vi "Main.vi"() -> ()   [LabVIEW 2017]
doc: "The myRIO Project template acquires acceleration data from the onboard accelerometer and displays the changes of acceleration values in a waveform chart."
uses:
  <vilib>/myRIO/Common/Instrument Driver Framework/myRIO v1.0/IRQ/typedefs/DI IRQ Type.ctl
  <vilib>/userdefined/High Color/nirio_resource_hc.ctl
  <vilib>/myRIO/Instrument Drivers/Onboard IO/DIO/typedefs/DIO Reference.ctl
  <vilib>/myRIO/Common/Instrument Driver Framework/Utilities/typedefs/myRIO Generic Hardware Reference.ctl
  <vilib>/myRIO/Common/Instrument Driver Framework/Utilities/typedefs/Hardware Version Enum.ctl
  <vilib>/myRIO/Common/Instrument Driver Framework/Utilities/typedefs/myRIO v1.0 Reference.ctl
  <vilib>/myRIO/Common/Instrument Driver Framework/Utilities/typedefs/Generic FPGA Reference.ctl
  <vilib>/myRIO/Common/Instrument Driver Framework/myRIO v1.0/DIO/typedefs/DIO Channels List.ctl
  <vilib>/myRIO/Common/Instrument Driver Framework/myRIO v1.0/DIO/typedefs/DIO Channels Enum.ctl
  <vilib>/myRIO/Common/Instrument Driver Framework/Utilities/vis/Is FPGA Ref Available.vi
  <vilib>/myRIO/Common/Instrument Driver Framework/myRIO v1.0/DIO/vis/myRIO v1.1 Open DIO.vi
  <vilib>/myRIO/Instrument Drivers/Onboard IO/DIO/vis/Write.vi
  <vilib>/myRIO/Common/Instrument Driver Framework/Utilities/vis/Validate Channels.vi
  <vilib>/myRIO/Common/Instrument Driver Framework/myRIO v1.0/DIO/vis/myRIO v1.0 Reserve DIO.vi
  <vilib>/myRIO/Common/Instrument Driver Framework/myRIO v1.0/Resource Manager/vis/myRIO v1.0 Reserve Channel List.vi
  <vilib>/myRIO/Common/Instrument Driver Framework/myRIO v1.0/DIO/vis/myRIO v1.0 Build MUX Configuration DIO.vi
  <vilib>/myRIO/Common/Instrument Driver Framework/myRIO v1.0/Resource Manager/vis/myRIO v1.0 Reserve Channel.vi
  <vilib>/myRIO/Common/Instrument Driver Framework/myRIO v1.0/Resource Manager/vis/myRIO v1.0 Unreserve Channel.vi
  <vilib>/myRIO/Common/Instrument Driver Framework/myRIO v1.0/Resource Manager/vis/myRIO v1.0 Create Configuration List.vi
  <vilib>/myRIO/Common/Instrument Driver Framework/myRIO v1.0/Resource Manager/vis/myRIO v1.0 Build Mutex Name.vi
  ACTION.vi
  SONG.vi
  <vilib>/myRIO/Common/Instrument Driver Framework/myRIO v1.0/IRQ/vis/myRIO v1.1 Register DI IRQ.vi
  <vilib>/Utility/VariantDataType/GetNumericInfo.vi
  <vilib>/Utility/error.llb/Error Cluster From Error Code.vi
  <vilib>/myRIO/Common/Instrument Driver Framework/myRIO v1.0/myRIO v1.1 Open.vi
  <vilib>/myRIO/Common/Instrument Driver Framework/Utilities/vis/IO Manager.vi
  <vilib>/myRIO/Common/Instrument Driver Framework/Utilities/vis/Configuration Manager.vi
  <vilib>/myRIO/Common/Instrument Driver Framework/myRIO v1.0/Resource Manager/vis/myRIO v1.0 Configure IO.vi
  <vilib>/myRIO/Common/Instrument Driver Framework/myRIO v1.0/myRIO v1.0 Close.vi
  <vilib>/myRIO/Common/Instrument Driver Framework/myRIO v1.0/DIO/vis/myRIO v1.0 Write DIO.vi
  <vilib>/myRIO/Instrument Drivers/IRQ/IO IRQ/vis/myRIO Register DI IRQ.xnode
  <vilib>/myRIO/Common/Instrument Driver Framework/myRIO v1.0/IRQ/typedefs/Callback VI Ref.ctl
  <vilib>/myRIO/Express VI/Onboard IO/DO/DO Express VI.xnode
  <vilib>/myRIO/Instrument Drivers/Onboard IO/DIO/vis/myRIO DIO Open.xnode
  <vilib>/myRIO/Instrument Drivers/Onboard IO/DIO/DIO.lvlib
panel:
  out "ACTION 2":string
  in  "Edge Count":u32=1
  out "SONG":string
  out "Gen Loop":i32
  out "inner loop":i32
  out "ACTION":string
  out "loop read":string
  in  "Stop Button":bool
  out "Selected Octave":i32[](array[numeric])
  out "Error Out 7":errorcluster
  in  "Error In 7":errorcluster
  out "Status":i32[](array[numeric])
  out "Number_of_elements in status":dbl
  out "Notes":i32[](array[numeric])
  out "Number_of_elements in notes":dbl
  out "Error Out 2":errorcluster
  in  "Error In 2":errorcluster
  out "Time":dbl[](array[numeric])
  out "Number_of_elements in time":dbl
  out "Error Out":errorcluster
  in  "Error In":errorcluster
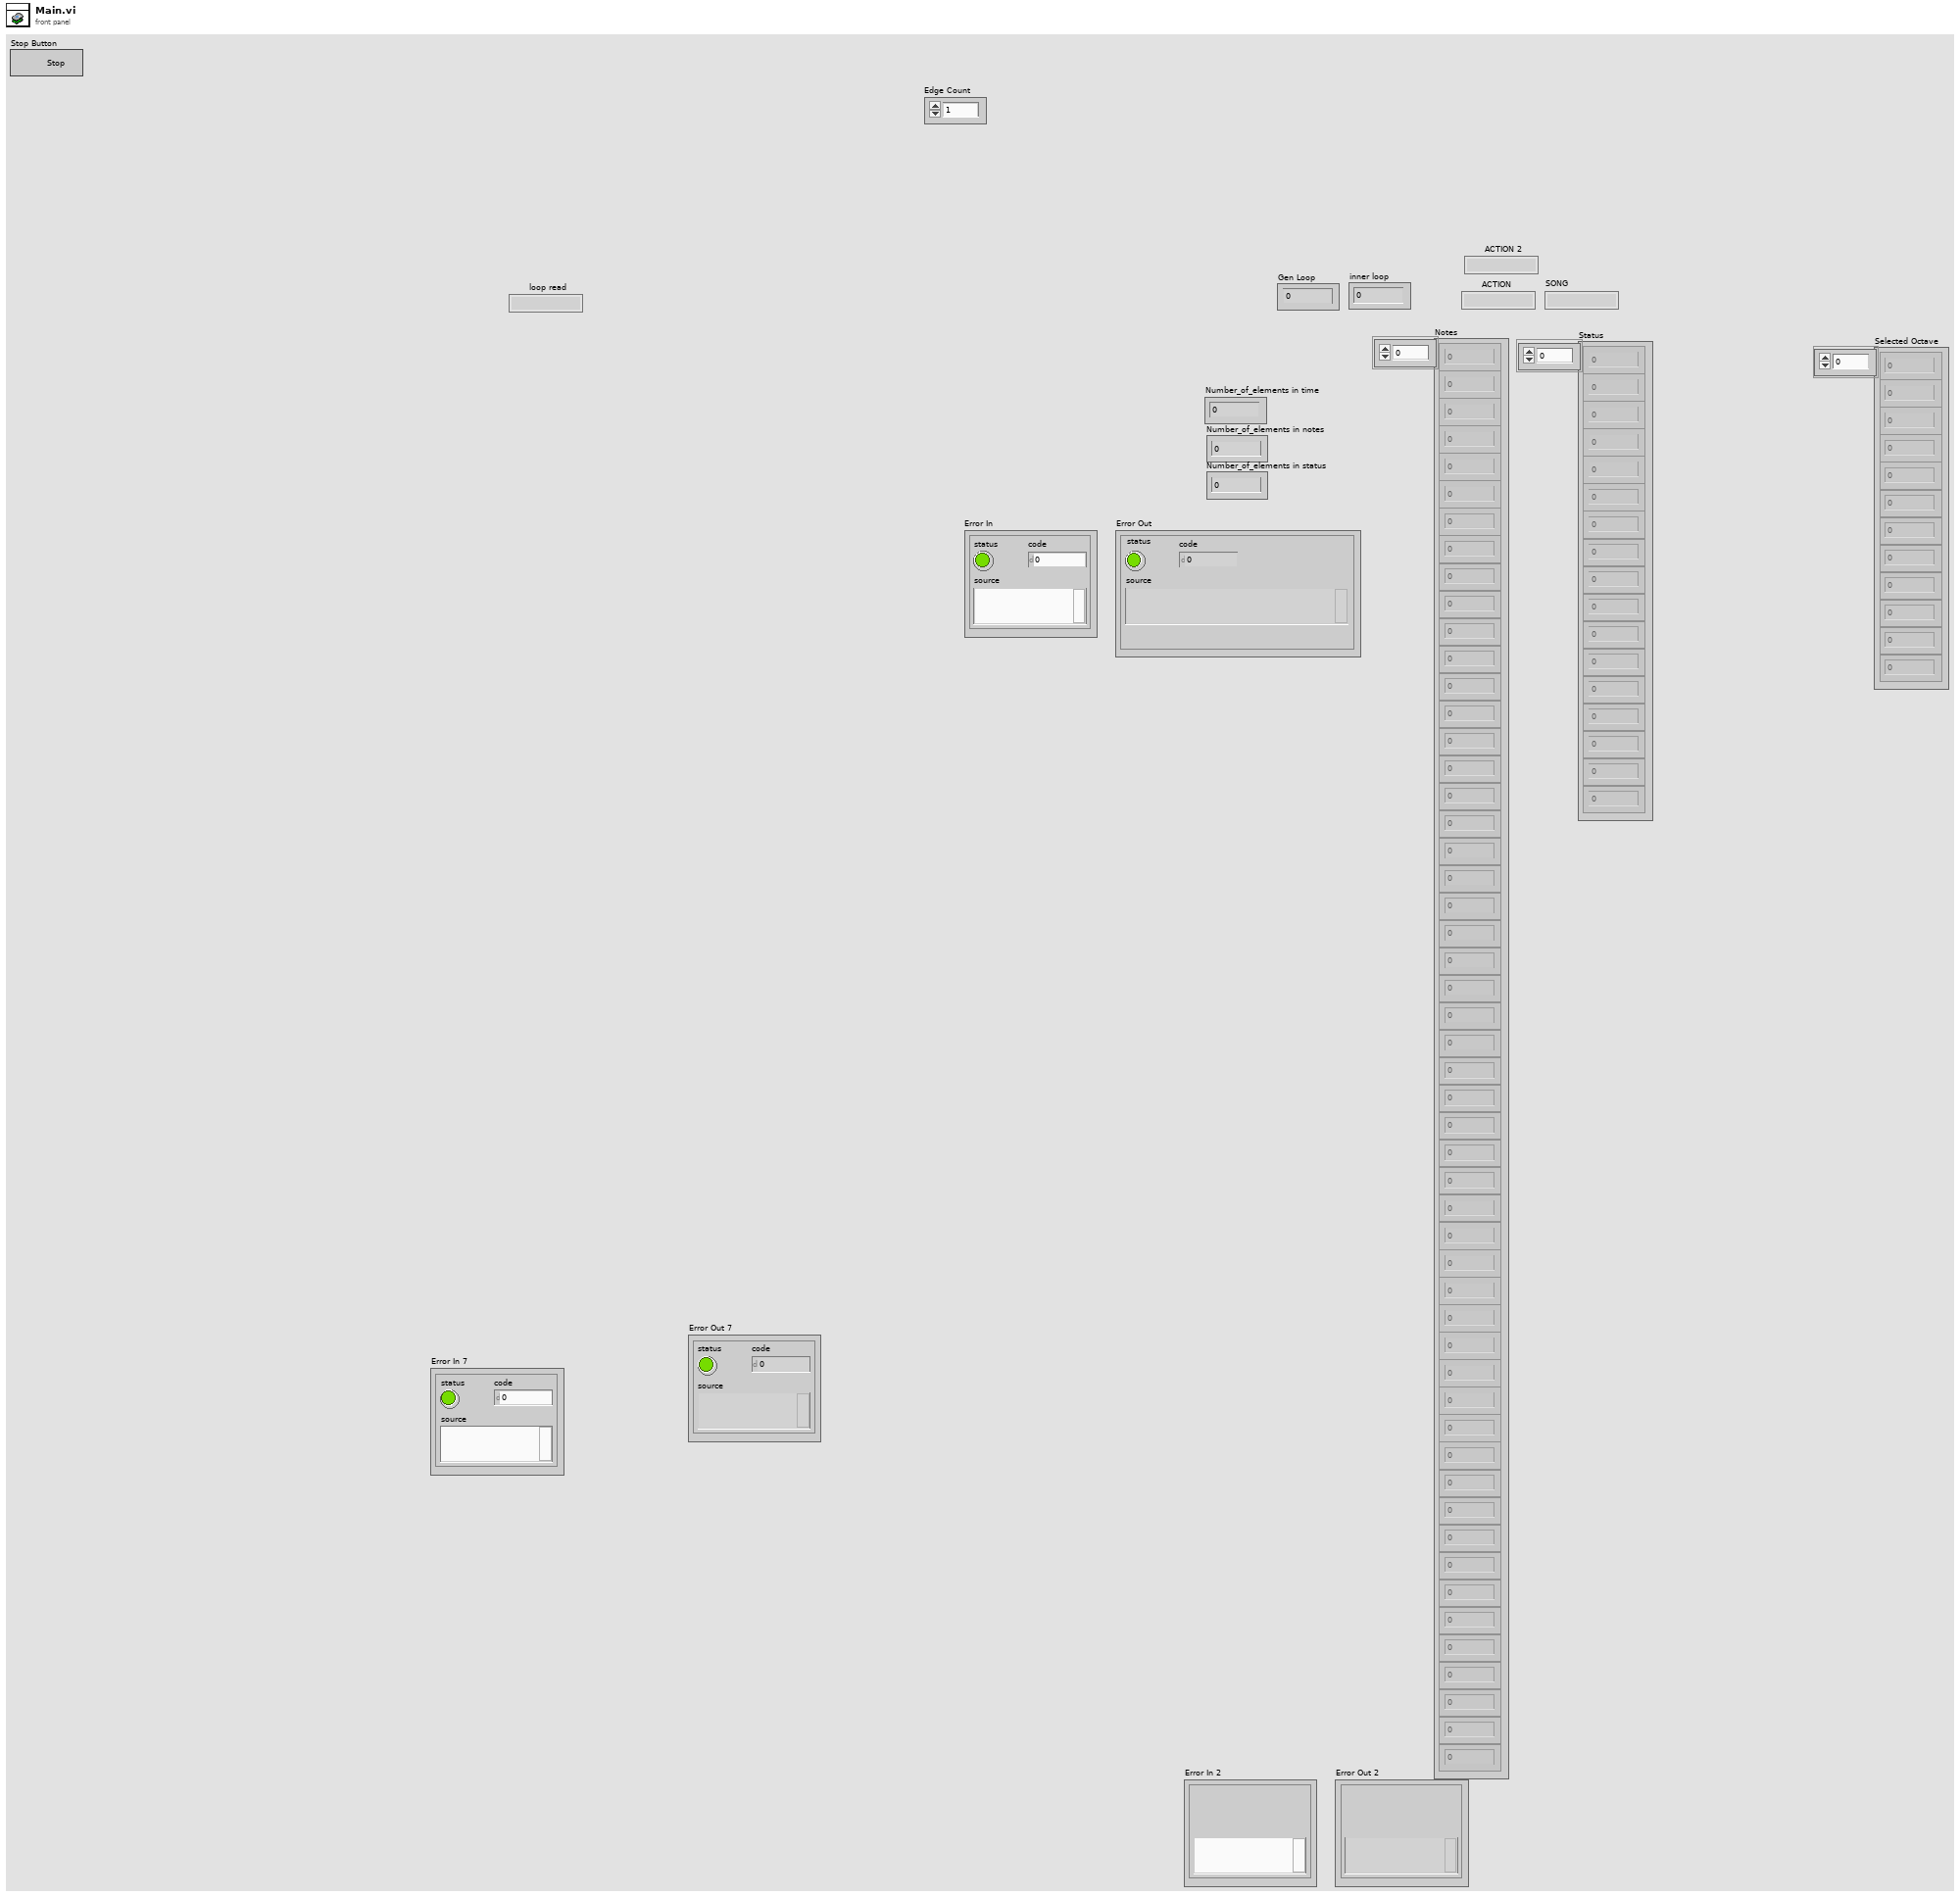
[diagram p1: front panel]
types:
  T1 = typedef "DI IRQ Type.ctl" = enum16{"Digital falling edge", "Digital rising edge", "Digital edge"}
  T2 = typedef "nirio_resource_hc.ctl" = tag
  T3 = typedef "DIO.lvlib/DIO Reference.ctl" = cluster{"myRIO Reference":T4, "DIO Channels List":T8}
  T4 = typedef "myRIO Generic Hardware Reference.ctl" = cluster{"myRIO Model":T5, "myRIO Hardware Reference":T6}
  T5 = typedef "Hardware Version Enum.ctl" = enum16{"Unknown", "myRIO-1900", "myRIO-1950", "roboRIO", "NI ELVIS RIO CM"}
  T6 = typedef "myRIO v1.0 Reference.ctl" = cluster{"Generic FPGA Reference":T7, "Allow multiple opens":bool}
  T7 = typedef "Generic FPGA Reference.ctl" = refnum<k20>
  T8 = typedef "DIO Channels List.ctl" = T9[]
  T9 = typedef "DIO Channels Enum.ctl" = enum16{"Not Connected", "C/DIO0", "C/DIO1", "C/DIO2", "C/DIO3", "C/DIO4", "C/DIO5", "C/DIO6", "C/DIO7", "A/DIO0", "A/DIO1", "A/DIO2", "A/DIO3", "A/DIO4", "A/DIO5", "A/DIO6", "A/DIO7", "A/DIO8", "A/DIO9", "A/DIO10", "A/DIO11", "A/DIO12", "A/DIO13", "A/DIO14", "A/DIO15", "B/DIO0", "B/DIO1", "B/DIO2", "B/DIO3", "B/DIO4", "B/DIO5", "B/DIO6", "B/DIO7", "B/DIO8", "B/DIO9", "B/DIO10", "B/DIO11", "B/DIO12", "B/DIO13", "B/DIO14", "B/DIO15", "LED0", "LED1", "LED2", "LED3", "Button0", "DIO/DIO0", "DIO/DIO1", "DIO/DIO2", "DIO/DIO3", "DIO/DIO4", "DIO/DIO5", "DIO/DIO6", "DIO/DIO7", "DIO/DIO8", "DIO/DIO9", "SPI/CS0", "SPI/CS1", "SPI/CS2", "SPI/CS3", "LED RADIO (Green)", "LED RADIO (Red)", "LED COMM (Green)", "LED COMM (Red)", "LED MODE (Green)", "LED MODE (Red)"}
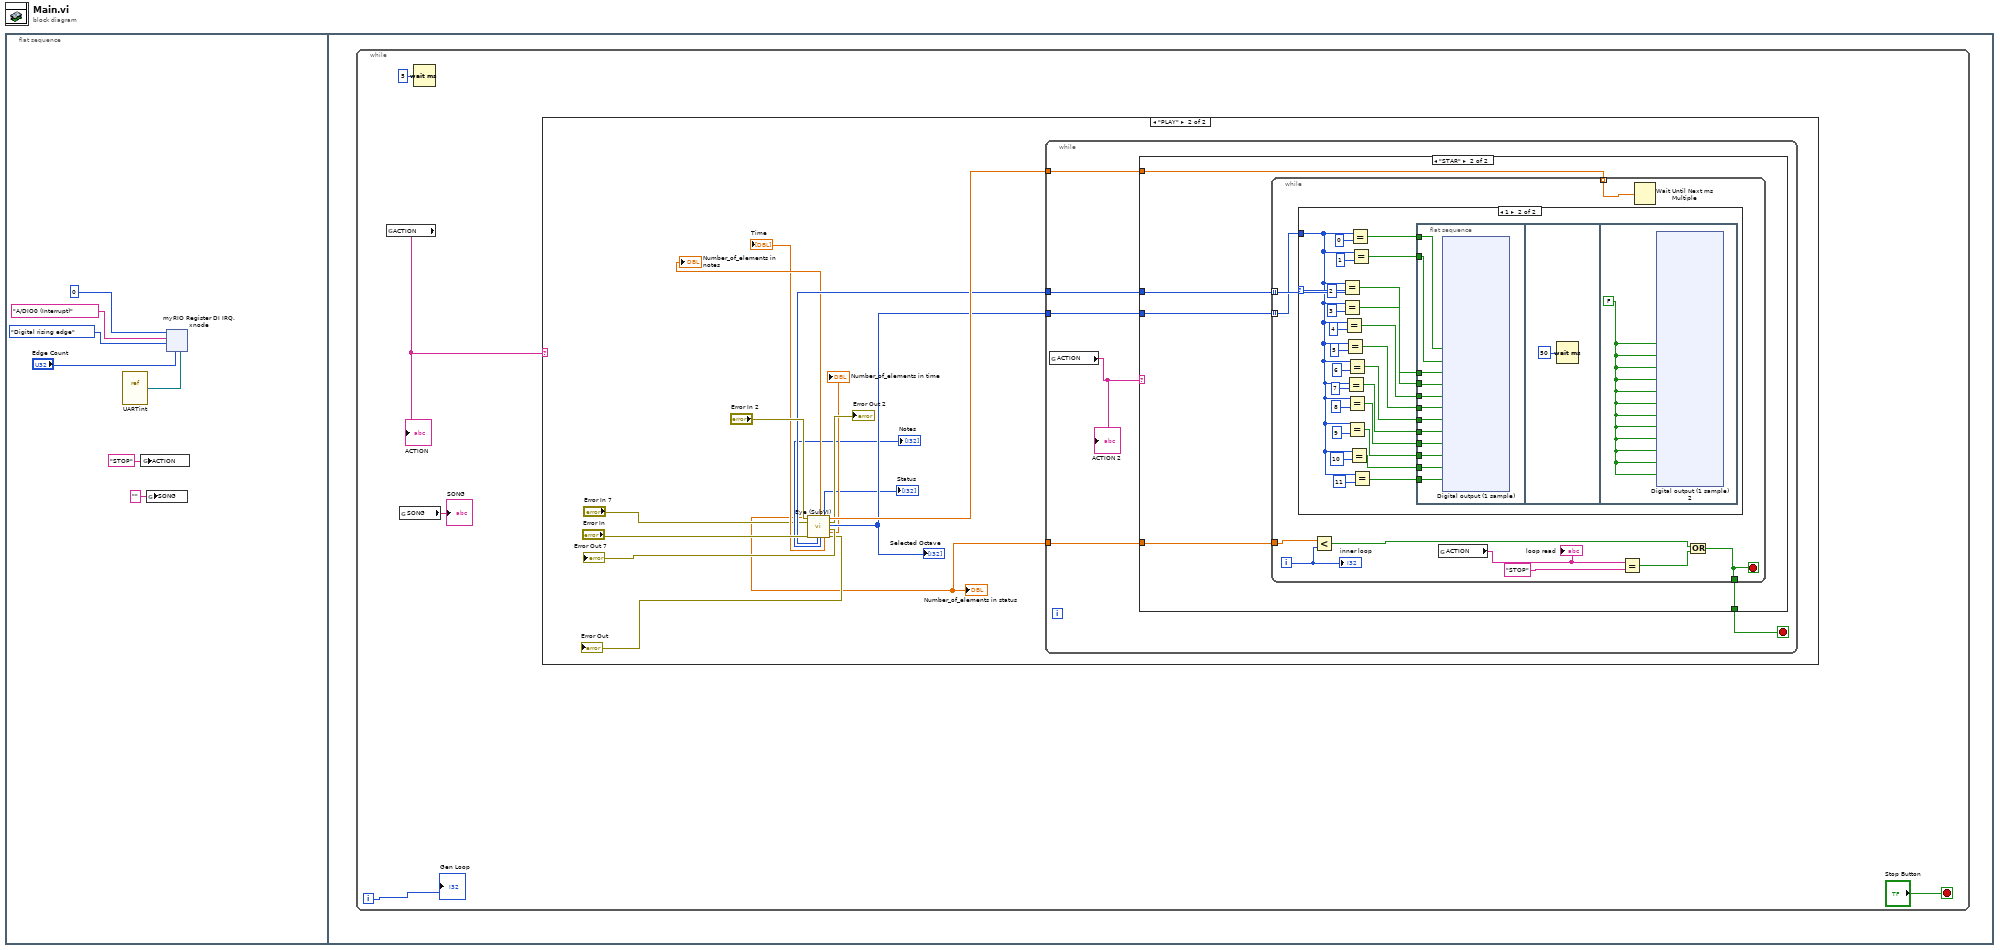
[diagram p0: block diagram]
diagram:
  n1 = flat-sequence {
    frame #0 {
      n2 = vi-ref "UARTint.vi"() -> ("vi reference"=w4:refnum<vi>)
      n3 = global write "ACTION.vi" "ACTION"("STOP" ("ACTION")) -> ()
      n4 = global write "SONG.vi" "SONG"("" ("SONG")) -> ()
      n5 = xnode "myRIO Register DI IRQ.xnode"("Channel Name"=tag "A/DIO0 (Interrupt)", "Callback VI Reference"=w4, "Edge Count"="Edge Count", "IRQ Number"=u8 0, "Digital Interrupt Type"=DI_IRQ_Type."Digital rising edge") -> ()  [unwired: 2 in, 1 out]
    }
    frame #1 {
      n6 = while {
        i -> [w18]
        stop <- "Stop Button" stop-if-true
        n7 = global read "ACTION.vi" "ACTION"() -> (w20:string)
        "ACTION" <- w20
        n8 = global read "SONG.vi" "SONG"() -> (→"SONG":string)
        n9 = Wait (ms)(milliseconds to wait=u32 5) -> ()  [unwired: 1 out]
        n10 = case shown="\"PLAY\"" w20 {
          frame "STOP", Default {
          }
          frame "PLAY" {
            n11 = call "Eye (SubVI).vi"("Error In in"="Error In 2", "Error In 7"="Error In 7", "error in (no error)"="Error In") -> ("Number_of_elements in status"=w22:dbl, "Array 2"=w33:i32[], "Number_of_elements in notes"=→"Number_of_elements in notes":dbl, "Notes"=→"Notes":i32[], "Status"=→"Status":i32[], "Time"=→"Time":dbl[], "Array 3"=w34:dbl[], "Error Out 2"=→"Error Out 2":errorcluster, "Array"=w32:i32[], "Error Out 7"=→"Error Out 7":errorcluster, "Number_of_elements in time"=→"Number_of_elements in time":dbl, "error out"=→"Error Out":errorcluster)  [unwired: 5 in]
            "Number_of_elements in status" <- w22
            "Selected Octave" <- w32
            n12 = while {
              tunnel: w34 -> [w42]
              tunnel: w33 -> [w41]
              tunnel: w32 -> [w40]
              tunnel: w22 -> [w38]
              stop <- w37 stop-if-true
              n13 = global read "ACTION.vi" "ACTION"() -> (w39:string)
              "ACTION 2" <- w39
              n14 = case shown="\"STAR\"" w39 {
                tunnel: w42 -> [_ w47]
                tunnel: w41 -> [_ w46]
                tunnel: w40 -> [_ w45]
                tunnel: w38 -> [_ w44]
                tunnel: [_ w43] -> w37
                frame Default {
                }
                frame "STAR" {
                  n15 = while {
                    tunnel: w45 -> [w56] mode=indexing
                    tunnel: w47 -> [w48] mode=indexing
                    tunnel: w46 -> [w57] mode=indexing
                    tunnel: w44 -> [w53]
                    tunnel: [w49] -> w43
                    i -> [w52]
                    stop <- w49 stop-if-true
                    n16 = case shown="1" w57 {
                      tunnel: w56 -> [_ w69]
                      frame 0, Default {
                      }
                      frame 1 {
                        n17 = Equal?(x=w69, y=2) -> (x = y?=w67:bool)
                        n18 = Equal?(x=w69, y=3) -> (x = y?=w66:bool)
                        n19 = Equal?(x=w69, y=4) -> (x = y?=w65:bool)
                        n20 = Equal?(x=w69, y=5) -> (x = y?=w64:bool)
                        n21 = Equal?(x=w69, y=7) -> (x = y?=w62:bool)
                        n22 = Equal?(x=w69, y=8) -> (x = y?=w61:bool)
                        n23 = Equal?(x=w69, y=6) -> (x = y?=w63:bool)
                        n24 = Equal?(x=w69, y=9) -> (x = y?=w60:bool)
                        n25 = Equal?(x=w69, y=10) -> (x = y?=w59:bool)
                        n26 = Equal?(x=w69, y=0) -> (x = y?=w81:bool)
                        n27 = Equal?(x=w69, y=1) -> (x = y?=w68:bool)
                        n28 = Equal?(x=w69, y=11) -> (x = y?=w58:bool)
                        n29 = flat-sequence {
                          tunnel: w81 -> [w94]
                          tunnel: w68 -> [w93]
                          tunnel: w67 -> [w92]
                          tunnel: w66 -> [w91]
                          tunnel: w65 -> [w90]
                          tunnel: w64 -> [w89]
                          tunnel: w63 -> [w88]
                          tunnel: w62 -> [w87]
                          tunnel: w61 -> [w83]
                          tunnel: w60 -> [w86]
                          tunnel: w59 -> [w85]
                          tunnel: w58 -> [w84]
                          frame #0 {
                            n30 = xnode "Digital output (1 sample)"("B/DIO0 (Pin 11)"=w94, "B/DIO1 (Pin 13)"=w93, "B/DIO2 (Pin 15)"=w92, "B/DIO3 (Pin 17)"=w91, "B/DIO4 (Pin 19)"=w90, "B/DIO5 (Pin 21)"=w89, "B/DIO6 (Pin 23)"=w88, "B/DIO7 (Pin 25)"=w87, "A/DIO7 (Pin 25)"=w83, "A/DIO1 (Pin 13)"=w86, "A/DIO2 (Pin 15)"=w85, "A/DIO3 (Pin 17)"=w84) -> ()  [unwired: 1 in, 1 out]
                          }
                          frame #1 {
                            n31 = Wait (ms)(milliseconds to wait=u32 50) -> ()  [unwired: 1 out]
                          }
                          frame #2 {
                            w142 = FALSE
                            n32 = xnode "Digital output (1 sample) 2"("B/DIO0 (Pin 11)"=w142, "B/DIO1 (Pin 13)"=w142, "B/DIO2 (Pin 15)"=w142, "B/DIO3 (Pin 17)"=w142, "B/DIO4 (Pin 19)"=w142, "B/DIO5 (Pin 21)"=w142, "B/DIO6 (Pin 23)"=w142, "B/DIO7 (Pin 25)"=w142, "A/DIO7 (Pin 25)"=w142, "A/DIO1 (Pin 13)"=w142, "A/DIO2 (Pin 15)"=w142, "A/DIO3 (Pin 17)"=w142) -> ()  [unwired: 1 in, 1 out]
                          }
                        }
                      }
                    }
                    n33 = Less?(x=w53, y=w52) -> (x < y?=w50:bool)
                    n34 = global read "ACTION.vi" "ACTION"() -> (w55:string)
                    "loop read" <- w55
                    n35 = Equal?(x=w55, y="STOP") -> (x = y?=w51:bool)
                    n36 = Wait Until Next ms Multiple(millisecond multiple=w48) -> ()  [unwired: 1 out]
                    n37 = Or(x=w50, y=w51) -> (x .or. y?=w49:bool)
                    "inner loop" <- w52
                  }
                }
              }
            }
          }
        }
        "Gen Loop" <- w18
      }
    }
  }
